vi "Initialize Hardware.vi"(8 "error in (no error)":errorcluster, 9 "Connection Ref":variant, 10 "DAQ Type":enum16{"Hardware", "Simulation"}(ring), 11 "AIT 429 in":refnum<class "AIT 429.lvclass">) -> (0 "error out":errorcluster, 3 "AIT 429 out":refnum<class "AIT 429.lvclass">)   [LabVIEW 2016, in "ARINC.lvlib" / "AIT 429.lvclass"]
uses:
  AIT 429.lvclass
  AIT 429.lvclass/AIT 429.ctl
  <instrlib>/AIT 429/Private/AIT 429 Initialize (Serial Number).vi
  <instrlib>/AIT 429/AIT 429.lvlib
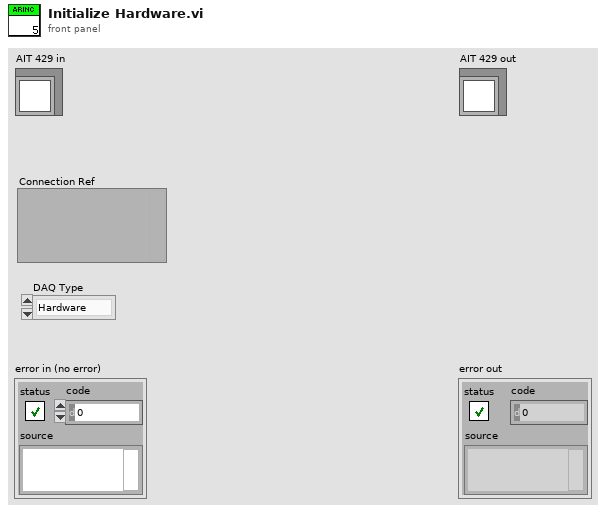
[diagram p1: front panel]
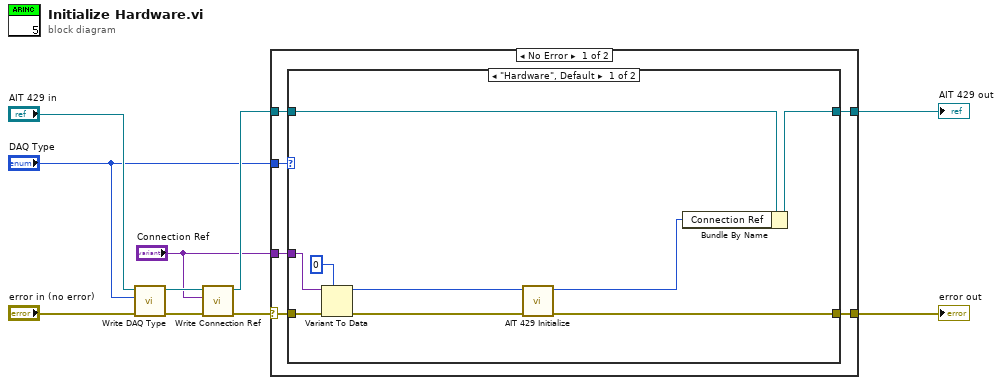
[diagram p0: block diagram]
diagram:
  n1 = call-dynamic "Write DAQ Type.vi"("error in (no error)"="error in (no error)", "DAQ Type"="DAQ Type", "AIT 429 in"="AIT 429 in") -> ("error out"=w9:errorcluster, "AIT 429 out"=w6:refnum<class "AIT 429.lvclass">)  [unwired: 7 in]
  n2 = call-dynamic "Write Connection Ref.vi"("error in (no error)"=w9, "Connection Ref"="Connection Ref", "AIT 429 in"=w6) -> ("error out"=w7:errorcluster, "AIT 429 out"=w5:refnum<class "AIT 429.lvclass">)  [unwired: 7 in]
  n3 = case shown="No Error" w7 {
    selector: w7 -> [w15 w28]
    tunnel: w5 -> [w13 w29]
    tunnel: "DAQ Type" -> [w16 _]
    tunnel: "Connection Ref" -> [w14 _]
    tunnel: [w12 w29] -> w2
    tunnel: [w11 w28] -> w1
    frame No Error {
      n4 = case shown="\"Hardware\", Default" w16 {
        tunnel: w15 -> [w25 w26]
        tunnel: w14 -> [w24 _]
        tunnel: w13 -> [w21 w27]
        tunnel: [w19 w27] -> w12
        tunnel: [w20 w26] -> w11
        frame "Hardware", Default {
          n5 = Variant To Data(error in=w25, type=u64 0 ("serial number"), Variant=w24) -> (data=w17:u64, error out=w23:errorcluster)
          n6 = call-poly <instrlib>:"AIT 429 Initialize.vi"("error in (no error)"=w23, "serial number"=w17) -> ("error out"=w20:errorcluster, "board handle"=w18:u32)  [unwired: 8 in]
          n7 = Bundle By Name(cluster=w21, "Connection Ref"=w18) -> (w19:refnum<class "AIT 429.lvclass">)
        }
        frame "Simulation" {
        }
      }
    }
    frame Error {
    }
  }
  "error out" <- w1
  "AIT 429 out" <- w2
